vi "Launcher.vi"   [LabVIEW 2020]
uses:
  HijodeDemo1/HijodeDemo1/HijodeDemo1.lvclass
  C:/Program Files (x86)/National Instruments/LabVIEW 2024/vi.lib/ActorFramework/Actor/Actor.lvclass
  <vilib>/ActorFramework/Actor/Actor.lvclass
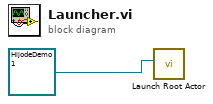
[diagram p0: block diagram]
diagram:
  n1 = call <vilib>:"Launch Root Actor.vi"("Actor"=refnum<class "HijodeDemo1.lvclass"> refnum ("HijodeDemo1.lvlib:HijodeDemo1.lvclass")) -> ()  [unwired: 9 in, 2 out]
